vi "Headers.vi"() -> (3 "Header Array OUT":string[](array[string]))   [LabVIEW 2018]
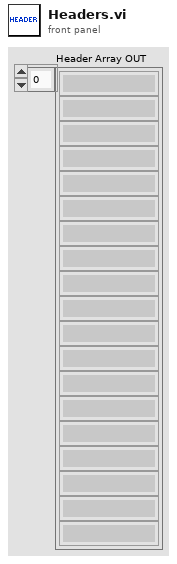
[diagram p1: front panel]
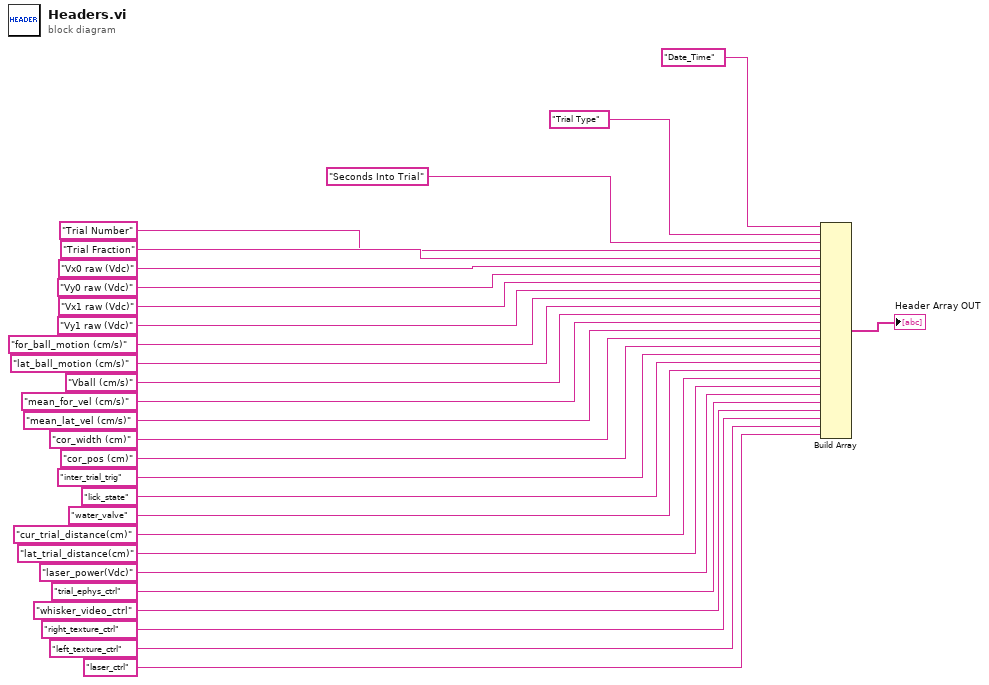
[diagram p0: block diagram]
diagram:
  n1 = Build Array("Date_Time" ("string"), "Trial Type" ("string"), "Seconds Into Trial" ("string"), "Trial Number" ("string"), "Trial Fraction" ("string"), "Vx0 raw (Vdc)" ("string"), "Vy0 raw (Vdc)" ("string"), "Vx1 raw (Vdc)" ("string"), "Vy1 raw (Vdc)" ("string"), "for_ball_motion (cm/s)" ("string"), "lat_ball_motion (cm/s)" ("string"), "Vball (cm/s)" ("string"), "mean_for_vel (cm/s)" ("string"), "mean_lat_vel (cm/s)" ("string"), "cor_width (cm)" ("string"), "cor_pos (cm)" ("string"), "inter_trial_trig" ("string"), "lick_state" ("string"), "water_valve" ("string"), "cur_trial_distance(cm)" ("string"), "lat_trial_distance(cm)" ("string"), "laser_power(Vdc)" ("string"), "trial_ephys_ctrl" ("string"), "whisker_video_ctrl" ("string"), "right_texture_ctrl" ("string"), "left_texture_ctrl" ("string"), "laser_ctrl" ("string")) -> (→"Header Array OUT":string[])
